vi "AlliGator Calibrate Single Phasor Plot.vi"(0 "Raw Phasor Plot":T6={"Phasor Plot Name"="", "Raw Phasor Plot"=[], "Phasor Frequency"=160000000.0, "[Decay Metadata]"=[], "Raw Phasor Plot SDV"=[], "Phasor SDV Options"={"Compute Estimated SDV"=FALSE, "# Replicas"=100, "Use Estimated Average Phasor"=FALSE}, "[Calibration Phasor]"=[]} {"[Decay Metadata]"."# Folds" min=1; "[Decay Metadata]"."ROI Descriptor"."Contours"."Type" items=["No Selection", "Point", "Line", "Rectangle", "Oval", "Polygon", "Freehand Region", "Annulus", "Unused2", "Unused3", "Broken Line", "Freehand Line", "Rotated Rectangle"]}, 5 "Calibration Phasor":T1, 7 "Calibration Phasor Series":T5, 9 "Phasor Calibration Map":T2={"Phasor Frequency"=80000000.0, "Calibration Lifetime"=1e-09, "ROI Centers"=[], "ROI Descriptors"=[], "Map Resolution X"=0, "Map Resolution Y"=0, "z Array"=[]} {"ROI Descriptors"."Contours"."Type" items=["No Selection", "Point", "Line", "Rectangle", "Oval", "Polygon", "Freehand Region", "Annulus", "Unused2", "Unused3", "Broken Line", "Freehand Line", "Rotated Rectangle"]}, 11 "Error In":errorcluster, 12 "Calibration Map MD5 Digest":string, 13 "Phasor Frequency":dbl[unit]) -> (4 "[Calibrated Phasor]":T4[](array[typedef]), 6 "# Recalibrated Phasors":i32, 8 "[Calibration Phasor]":T1[](array[typedef]), 15 "Error Out":errorcluster)   [LabVIEW 2021, in "AlliGator Phasor Calibration.lvlib"]
doc: "Applies phasor calibration to a single phasor plot.\n\nTakes into account whether a single phasor calibration, a phasor map or a phasor calibration series is used.\n\nFor a calibration map, takes into account the location of each individual phasor in the phasor plot."
uses:
  AlliGator Phasor Calibration.lvlib
  AlliGator Raw Phasor Plot Data v4.ctl
  Phasor/Phasor (g, s).ctl
  AlliGator Decay Metadata v3.ctl
  AlliGator Decay Background Subtraction Info.ctl
  AlliGator Baseline Subtraction Method.ctl
  Graphs/XY Graph/XY Graph Plot Shift Parameters.ctl
  Graphs/XY Graph/XY Graph Plot Shift Method.ctl
  AlliGator Decay Extrapolation Parameters.ctl
  Phasor/Phasor Standard Deviation Options.ctl
  Phasor/Calibration Phasor (m, phi).ctl
  Phasor/Phasor Reference Series.ctl
  Phasor/Phasor Calibration Map v2.ctl
  AlliGator Settings List.ctl
  Phasor/Phasor Calibration Type.ctl
  Utilities/Utilities.lvlib
  Phasor/Phasor.lvlib
  AlliGator Settings.lvlib
  AlliGator Phasor Graph.lvlib
  AlliGator Decay Preprocessing.lvlib
  Graphs/XY Graph/XY Graph Add-Ons.lvlib
panel:
  # "see the AlliGator License on the block diagram (Ctrl+E or Window:Show Block Diagram)"
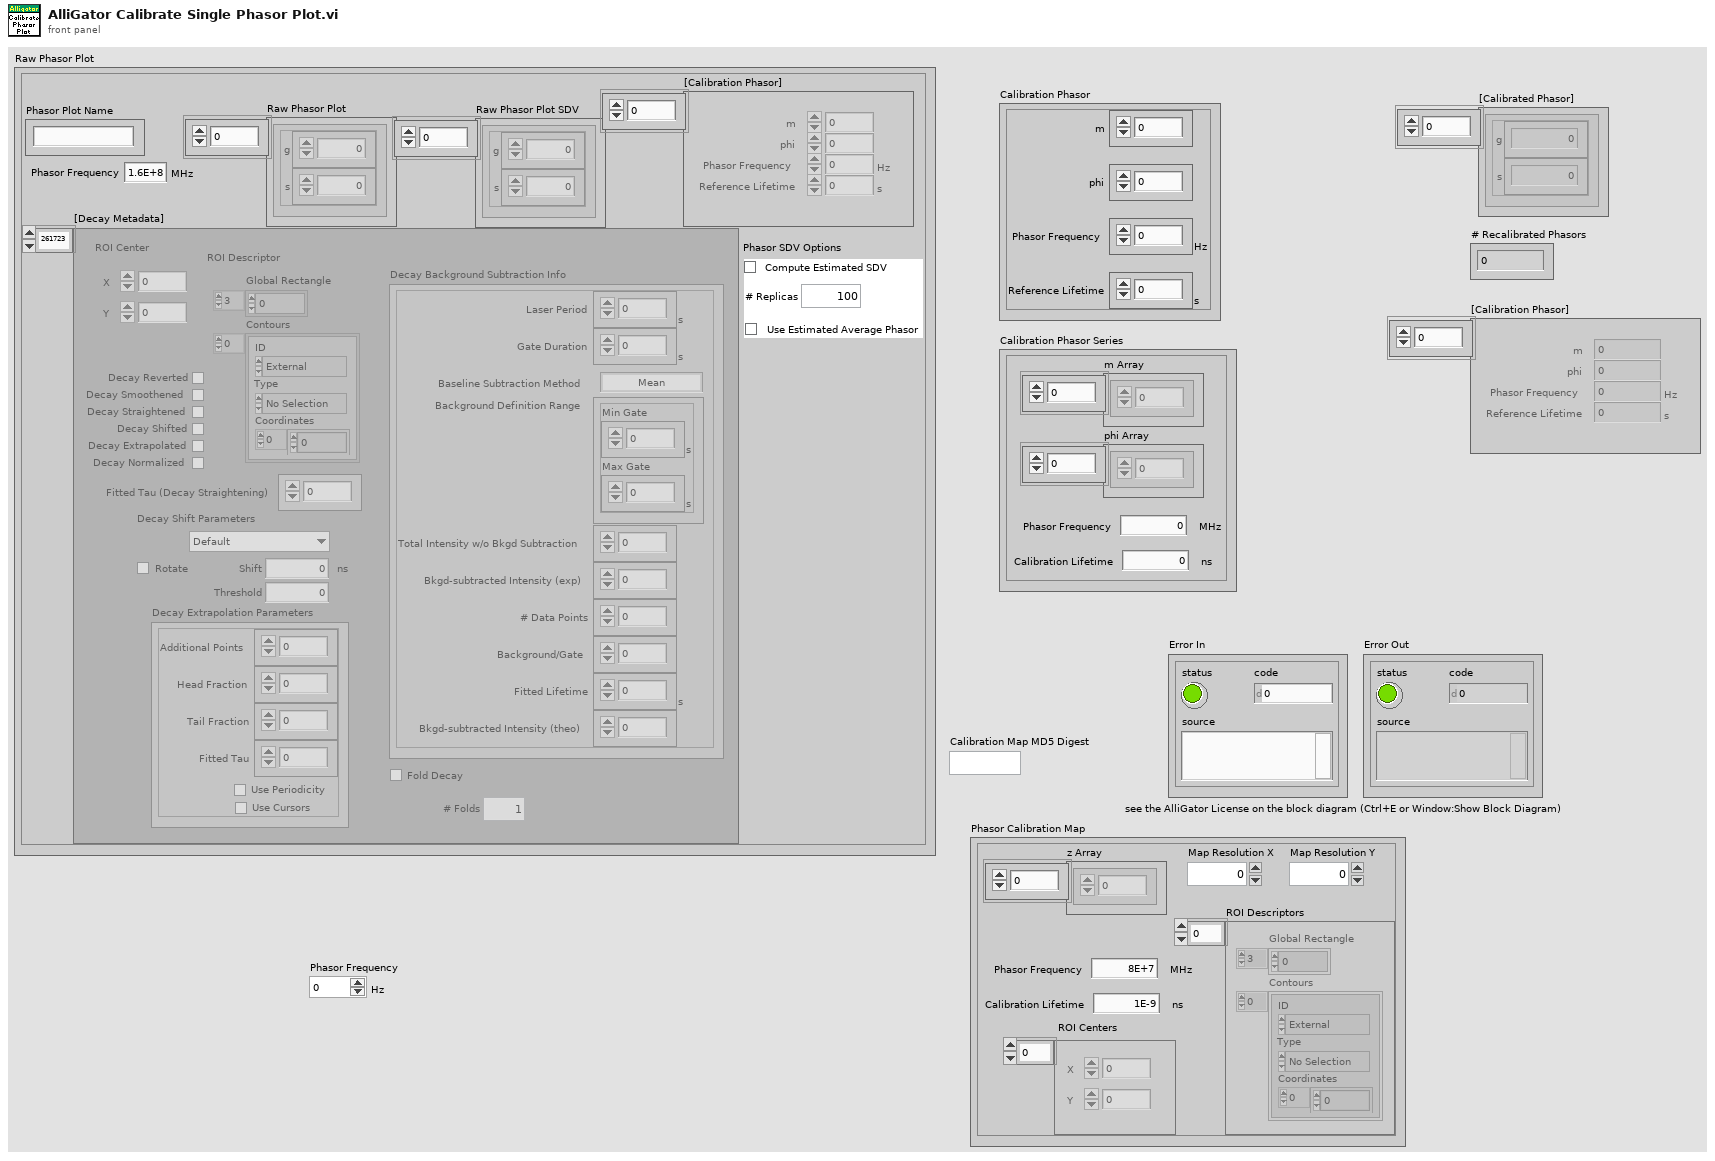
[diagram p1: front panel]
types:
  T1 = typedef "Phasor.lvlib/Calibration Phasor (m, phi).ctl" = cluster{"m":dbl, "phi":dbl, "Phasor Frequency":dbl[unit], "Reference Lifetime":dbl[unit]}
  T2 = typedef "Phasor.lvlib/Phasor Calibration Map v2.ctl" = cluster{"Phasor Frequency":dbl[unit], "Calibration Lifetime":dbl[unit], "ROI Centers":cluster{"X":i32, "Y":i32}[], "ROI Descriptors":T3[], "Map Resolution X":i32, "Map Resolution Y":i32, "z Array":cdb[]}
  T3 = typedef "ROI Descriptor" = cluster{"Global Rectangle":i32[], "Contours":cluster{"ID":enum32{"External", "Internal"}, "Type":u32, "Coordinates":i32[]}[]}
  T4 = typedef "Phasor.lvlib/Phasor (g, s).ctl" = cluster{"g":dbl, "s":dbl}
  T5 = typedef "Phasor.lvlib/Phasor Reference Series.ctl" = cluster{"m Array":dbl[], "phi Array":dbl[], "Phasor Frequency":dbl[unit], "Calibration Lifetime":dbl[unit]}
  T6 = typedef "AlliGator Phasor Graph.lvlib/AlliGator Raw Phasor Plot Data v4.ctl" = cluster{"Phasor Plot Name":string, "Raw Phasor Plot":T4[], "Phasor Frequency":dbl[unit], "[Decay Metadata]":T7[], "Raw Phasor Plot SDV":T4[], "Phasor SDV Options":T13, "[Calibration Phasor]":T1[]}
  T7 = typedef "AlliGator Phasor Graph.lvlib/AlliGator Decay Metadata v3.ctl" = cluster{"ROI Descriptor":T3, "ROI Center":cluster{"X":i32, "Y":i32}, "Decay Background Subtraction Info":T8, "Decay Reverted":bool, "Decay Smoothened":bool, "Decay Straightened":bool, "Fitted Tau (Decay Straightening)":dbl, "Decay Shift Parameters":T10, "Decay Shifted":bool, "Decay Extrapolated":bool, "Decay Extrapolation Parameters":T12, "Decay Normalized":bool, "Fold Decay":bool, "# Folds":u32}
  T8 = typedef "AlliGator Decay Analysis.lvlib/AlliGator Decay Preprocessing.lvlib/AlliGator Decay Background Subtraction Info.ctl" = cluster{"Laser Period":dbl[unit], "Gate Duration":dbl[unit], "Baseline Subtraction Method":T9, "Background Definition Range":cluster{"Min Gate":dbl[unit], "Max Gate":dbl[unit]}, "Total Intensity w/o Bkgd Subtraction":dbl, "Bkgd-subtracted Intensity (exp)":dbl, "# Data Points":i32, "Background/Gate":dbl, "Fitted Lifetime":dbl[unit], "Bkgd-subtracted Intensity (theo)":dbl}
  T9 = typedef "AlliGator Decay Analysis.lvlib/AlliGator Decay Preprocessing.lvlib/AlliGator Baseline Subtraction Method.ctl" = enum16{"Mean", "Min", "Square Gated Single-Exponential", "File", "Constant"}
  T10 = typedef "XY Graph Add-Ons.lvlib/XY Graph Plot Shift Parameters.ctl" = cluster{"Type":T11, "Shift":dbl[unit], "Threshold":dbl, "Rotate":bool}
  T11 = typedef "XY Graph Add-Ons.lvlib/XY Graph Plot Shift Method.ctl" = enum16{"Default", "CFD", "Threshold", "Cross-Correlation"}
  T12 = typedef "AlliGator Decay Analysis.lvlib/AlliGator Decay Preprocessing.lvlib/AlliGator Decay Extrapolation Parameters.ctl" = cluster{"Additional Points":u32, "Head Fraction":dbl, "Fitted Tau":dbl, "Use Periodicity":bool, "Use Cursors":bool, "Tail Fraction":dbl}
  T13 = typedef "Phasor.lvlib/Phasor Standard Deviation Options.ctl" = cluster{"Compute Estimated SDV":bool, "# Replicas":u32, "Use Estimated Average Phasor":bool}
  T14 = typedef "Phasor.lvlib/Phasor Calibration Type.ctl" = enum16{"None", "Single Phasor", "Phasor Series", "Phasor Map"}
  T15 = typedef "AlliGator Settings.lvlib/AlliGator Settings List.ctl" = enum16{"GUI:Visible Settings Tab", "GUI:Last Run Version", "Source Image:Use Image Histogram for Contrast", "Source Image:Low Count Pixels Rejection Options", "Source Image:High Count Pixels Rejection Options", "Source Image:Use Image Brightness", "Source Image:Blend Overlay with Image Background", "Source Image:Use Fixed ROI Diameter", "Source Image:ROI Diameter", "Source Image:ROI Center Color", "Source Image:Peak Threshold", "Source Image:Intensity Threshold", "Source Image:Image Binning Options", "Source Image:Image Smoothing Options", "Source Image:Image Histogram Active", "Source Image:Invert Binary Mask", "Source Image:Hot Pixel Removal", "Source Image:Overlay Analyzed ROI Center", "Source Image:Auto-Adjust Contrast", "Source Image:Histogram Lower Percentile", "Source Image:Histogram Upper Percentile", "Source Image:Save Source Image", "Source Image:Scale Bar Options", "Source Image:Image Resolution (Pixel Size)", "Source Image:Flatfield Correction", "Source Image:Show Dead Left Columns Correction", "Source Image:Dead Left Columns Correction", "Source Image:Image Pre-Processing Operations Order", "Data Information:Gate Width", "Data Information:Nanotime Gate Separation", "Data Information:Macrotime Gate Separation", "Data Information:Gate Step", "Data Information:# Gates", "Data Information:Gate Image Exposure", "Data Information:Gate Image Integration", "Data Information:Gates to Skip", "Data Information:Gates to Keep", "Data Information:Define Gates to", "Data Information:Channel Name", "Data Information:Available Channel Names", "Data Information:Channel Arithmetic", "Data Information:Background File Subtraction", "Data Information:Background File", "Data Information:Background Scaling Factor", "Data Information:Background Pile-up Correction", "Data Information:Background Pixel Well Capacity", "Data Information:Laser Period", "Data Information:SYNC Period", "Data Information:Pile-up Correction", "Data Information:Pixel Well Capacity", "Data Information:Dataset Scaling Factor", "Fluorescence Decay_Decay Pre-Processing:Reverse Gates", "Fluorescence Decay_Decay Pre-Processing:Verbose Decay Pre-Processing", "Fluorescence Decay_Decay Pre-Processing:Use Decay Pre-Processing", "Fluorescence Decay_Decay Pre-Processing:Background Subtraction", "Fluorescence Decay_Decay Pre-Processing:Background Definition Range", "Fluorescence Decay_Decay Pre-Processing:Baseline Subtraction Method", "Fluorescence Decay_Decay Pre-Processing:Decay Pre-Processing Operations Order", "Fluorescence Decay_Decay Pre-Processing:Smoothing Parameter", "Fluorescence Decay_Decay Pre-Processing:Shift Decay", "Fluorescence Decay_Decay Pre-Processing:Decay Shift Parameters", "Fluorescence Decay_Decay Pre-Processing:Fold Decay", "Fluorescence Decay_Decay Pre-Processing:# Folds", "Fluorescence Decay_Decay Pre-Processing:1-Normalize Decay", "Fluorescence Decay_Decay Pre-Processing:[0-1]-Normalize Decay", "Fluorescence Decay_Decay Pre-Processing:Smoothen Decay", "Fluorescence Decay_Decay Pre-Processing:Extrapolate Decay", "Fluorescence Decay_Decay Pre-Processing:Use Periodicity", "Fluorescence Decay_Decay Pre-Processing:Use Cursors", "Fluorescence Decay_Decay Pre-Processing:Tail Fraction", "Fluorescence Decay_Decay Pre-Processing:Head Fraction", "Fluorescence Decay_Decay Pre-Processing:Additional Points", "Fluorescence Decay_Decay Pre-Processing:Straighten Decay", "Fluorescence Decay_Decay Pre-Processing:Constant Background", "Fluorescence Decay_Decay Pre-Processing:Pixel-Normalize Decay", "Fluorescence Decay_Advanced Analysis:Extract IRF instead of Decay", "Fluorescence Decay_Advanced Analysis:IRF Extraction Options", "Fluorescence Decay_Advanced Analysis:IRF Optimization Options", "Fluorescence Decay_Advanced Analysis:Square Pulse Options", "Fluorescence Decay_Advanced Analysis:IRF Order", "Fluorescence Decay_Advanced Analysis:IRF Time Constants", "Fluorescence Decay_Advanced Analysis:Wavelet Analysis Options", "Fluorescence Decay_Advanced Analysis:Average Lifetime Options", "Fluorescence Decay_Fit Options:Fit Options", "Fluorescence Decay_Fit Options:Use Legacy Fitting Approach", "Fluorescence Decay_Fit Options:Use Data Information Laser Period", "Fluorescence Decay_Fit Parameters:Displayed Fit Parameters", "Fluorescence Decay_Fit Parameters:Fit Parameter Constraints", "Fluorescence Decay_Fit Parameters:Export Tabulated Results", "Fluorescence Decay_Fit Parameters:MLE Baseline Offset Type", "Fluorescence Decay_Fit Parameters:MLE Baseline Offset", "Fluorescence Decay_Fit Parameters:Guess Parameter Names", "Fluorescence Decay_Fit Parameters:Guess Parameter Values", "Fluorescence Decay_Fit Parameters:Guess Parameters Options", "Fluorescence Decay_Styles:Show Last Decay Only", "Fluorescence Decay_Styles:Decay Graph Color Array", "Fluorescence Decay:Decay Graph Active", "Fluorescence Decay Statistics:Min Peak Value", "Fluorescence Decay Statistics:Reject Low Decay Peak Pixels", "Fluorescence Decay Statistics:Reject High Decay Peak Pixels", "Fluorescence Decay Statistics:Max Peak Value", "Time Traces:Use File Timestamp", "Time Traces:Time Step", "Time Traces:Use Intensity Correction File", "Time Traces:Intensity Correction File", "Phasor Plot:Phasor Plot Smoothing Options", "Phasor Plot:Phasor Plot Size", "Phasor Plot:Phasor Plot Graphics Options", "Phasor Plot:Cumulative Phasor Plot", "Phasor Plot:Use Phasor Brightness", "Phasor Plot:Blend Overlay with Phasor Background", "Phasor Plot:Save Phasor Plot", "Phasor Plot:Show References", "Phasor Plot:Phasor Ratio Decay Range", "Phasor Plot:Exponential Fading", "Phasor Plot:Phasor Ratio Reference Colors", "Phasor Plot:Reference Radius", "Phasor Plot:Show Color Map Vertices", "Phasor Plot:Phasor Plot Active", "Phasor Plot:Phasor Ratio Color Map Type", "Phasor Plot:Phasor Ratio Color Map", "Phasor Plot:Phasor Ratio Display Range", "Phasor Plot:Selected Image ROI(s)", "Phasor Plot:All Image ROIs", "Phasor Plot:Selected Phasor Plot ROI(s)", "Phasor Plot:All Phasor Plot ROIs", "Phasor Plot:Phasor Ratio Color-Coded Quantity", "Phasor Plot:Store Phasor Harmonics", "Phasor Plot:Draw Reference Segment", "Phasor Plot:User-Defined Quantity", "Phasor Graph:Phasor Frequency", "Phasor Graph:Phasor Ratio Type", "Phasor Graph:Pixel-level Phasor Computation", "Phasor Graph:Save Phasor Graph", "Phasor Graph:Phasor Graph Active", "Phasor Graph:Phasor SDV Options", "Phasor Calibration:Use Backup Calibration if needed", "Phasor Graph:Define Shortest Lifetime as", "Phasor Calibration:Backup Calibration Type", "Phasor Calibration:Calibration Type", "Phasor Calibration:Calibration Lifetime", "Phasor Calibration:Calibration Map Algorithm", "Single-Exponential Phasor Locus (SEPL):Gate Parameters", "Single-Exponential Phasor Locus (SEPL):User-defined Gate", "Single-Exponential Phasor Locus (SEPL):User-defined IRF", "Single-Exponential Phasor Locus (SEPL):Phasor Parameters", "Single-Exponential Phasor Locus (SEPL):Decay & IRF Parameters", "Single-Exponential Phasor Locus (SEPL):Display Parameters", "Lifetime Analysis:Decay Analysis Parameters", "Lifetime Analysis:Lifetime Map Active", "Plugins:Python Settings", "Miscellaneous:Verbose Mode", "Miscellaneous:Beep after Script", "Miscellaneous:Saved Image File Format", "Miscellaneous:Exported Gate Image Settings", "Miscellaneous:Include Loading in Timing", "Miscellaneous:Verbose Settings Mode", "Miscellaneous:Histogram Options", "Miscellaneous:Beep on Error", "Miscellaneous:# Logical Processors Used", "Miscellaneous:ROI Description Max Characters", "Miscellaneous:Verbose Error Mode", "Miscellaneous:Transparent Mask Color"}
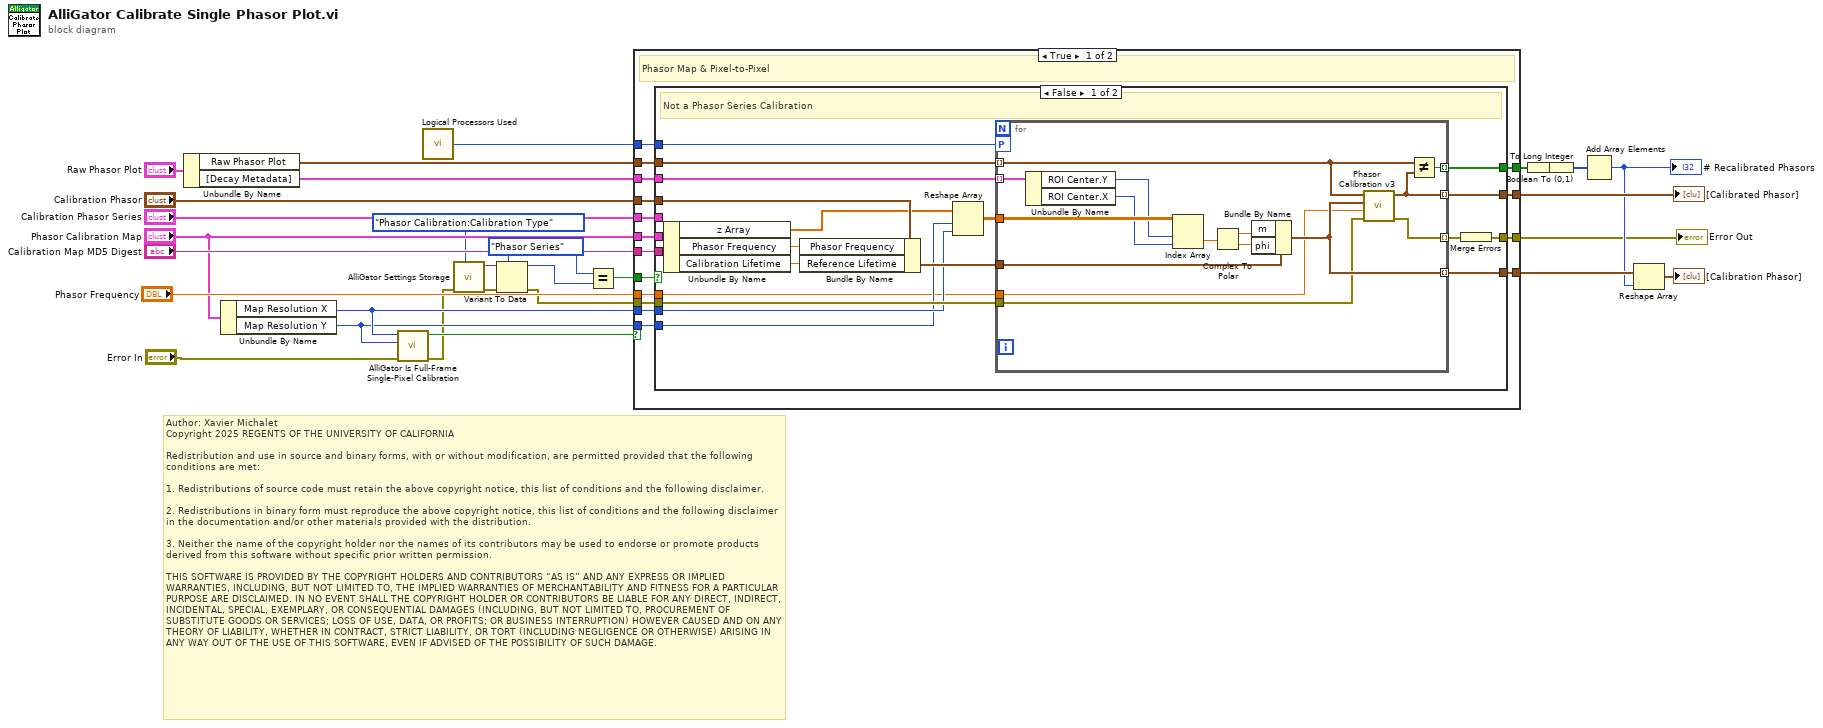
[diagram p0: block diagram]
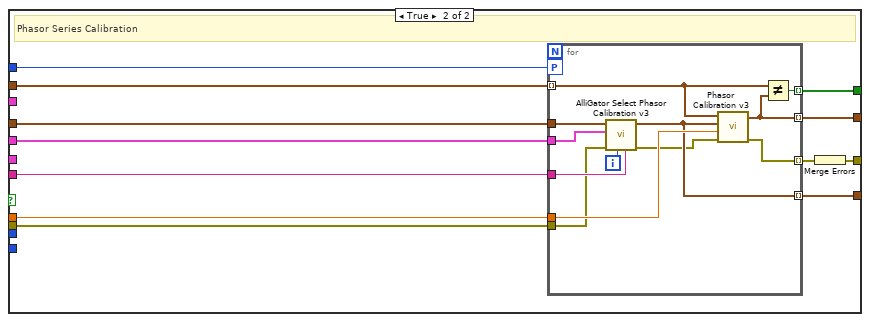
[diagram p2: hidden frame]
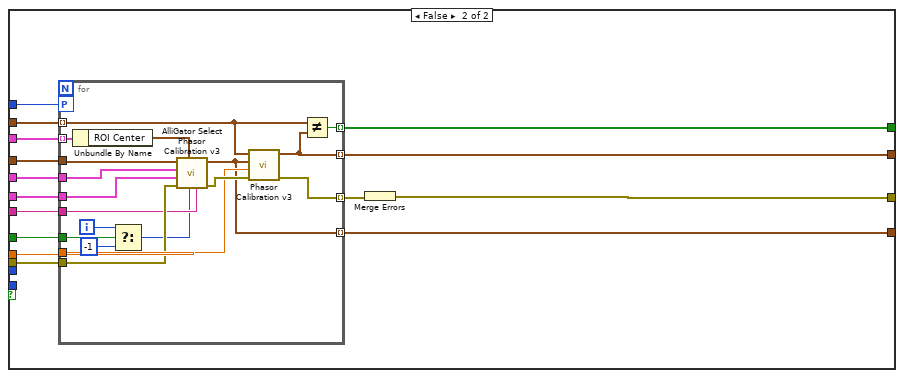
[diagram p3: hidden frame]
diagram:
  w2 = Phasor_Calibration_Type."Phasor Series" ("Calibration Type")
  # "Author: Xavier Michalet\nCopyright 2025 REGENTS OF THE UNIVERSITY OF CALIFORNIA\n\nRedistribution and use in source and binary forms, with or without modification, are permitted provided that the following conditions are met:\n\n1. Redistributions of source code must retain the above copyright notice, this list of conditions and the following disclaimer.\n\n2. Redistributions in binary form must reproduce the above copyright notice, this list of conditions and the following disclaimer in the documentation and/or other materials provided with the distribution.\n\n3. Neither the name of the copyright holder nor the names of its contributors may be used to endorse or promote products derived from this software without specific prior written permission.\n\nTHIS SOFTWARE IS PROVIDED BY THE COPYRIGHT HOLDERS AND CONTRIBUTORS “AS IS” AND ANY EXPRESS OR IMPLIED WARRANTIES, INCLUDING, BUT NOT LIMITED TO, THE IMPLIED WARRANTIES OF MERCHANTABILITY AND FITNESS FOR A PARTICULAR PURPOSE ARE DISCLAIMED. IN NO EVENT SHALL THE COPYRIGHT HOLDER OR CONTRIBUTORS BE LIABLE FOR ANY DIRECT, INDIRECT, INCIDENTAL, SPECIAL, EXEMPLARY, OR CONSEQUENTIAL DAMAGES (INCLUDING, BUT NOT LIMITED TO, PROCUREMENT OF SUBSTITUTE GOODS OR SERVICES; LOSS OF USE, DATA, OR PROFITS; OR BUSINESS INTERRUPTION) HOWEVER CAUSED AND ON ANY THEORY OF LIABILITY, WHETHER IN CONTRACT, STRICT LIABILITY, OR TORT (INCLUDING NEGLIGENCE OR OTHERWISE) ARISING IN ANY WAY OUT OF THE USE OF THIS SOFTWARE, EVEN IF ADVISED OF THE POSSIBILITY OF SUCH DAMAGE."
  n1 = Unbundle By Name("Raw Phasor Plot") -> ("Raw Phasor Plot"=w25:T4[], "[Decay Metadata]"=w24:T7[])
  n2 = Unbundle By Name("Phasor Calibration Map") -> ("Map Resolution X"=w14:i32, "Map Resolution Y"=w11:i32)
  n3 = call "AlliGator Is Full-Frame Single-Pixel Calibration.vi"("error in (no error)"="Error In", "Map Resolution Y"=w11, "Map Resolution X"=w14) -> ("error out"=w5:errorcluster, "Full-Frame Single-Pixel Calibration?"=w12:bool)  [unwired: 7 in]
  n4 = call "Logical Processors Used.vi"() -> ("# Logical Processor Used"=w10:i32)  [unwired: 6 in]
  n5 = call "AlliGator Settings Storage.vi"("AlliGator Settings List"=AlliGator_Settings_List."Phasor Calibration:Calibration Type", "Error In"=w5) -> ("Error Out"=w6:errorcluster, "Variant Data out"=w7:variant)  [unwired: 8 in]
  n6 = Variant To Data(error in=w6, type=w2, Variant=w7) -> (data=w3:T14, error out=w4:errorcluster)
  n7 = Equal?(x=w2, y=w3) -> (x = y?=w1:bool)
  n8 = case shown="True" w12 {
    tunnel: "Calibration Phasor" -> [w39 w118]
    tunnel: "Calibration Phasor Series" -> [w31 w117]
    tunnel: [w45 w116] -> w26
    tunnel: w25 -> [w44 w115]
    tunnel: "Phasor Calibration Map" -> [w43 w114]
    tunnel: w24 -> [w42 w113]
    tunnel: "Calibration Map MD5 Digest" -> [w30 w112]
    tunnel: [w41 w111] -> w22
    tunnel: "Phasor Frequency" -> [w33 w110]
    tunnel: [w40 w109] -> w18
    tunnel: w4 -> [w38 w108]
    tunnel: w14 -> [w37 _]
    tunnel: w11 -> [w36 _]
    tunnel: w10 -> [w35 w107]
    tunnel: [w34 w105] -> w9
    tunnel: w1 -> [w32 w104]
    frame True {
      # "Phasor Map & Pixel-to-Pixel"
      n9 = case shown="False" w32 {
        tunnel: [w64 w91] -> w45
        tunnel: w44 -> [w63 w90]
        tunnel: w43 -> [w62 _]
        tunnel: w42 -> [w61 _]
        tunnel: [w60 w89] -> w41
        tunnel: [w59 w88] -> w40
        tunnel: w39 -> [w58 w81]
        tunnel: w38 -> [w55 w87]
        tunnel: w37 -> [w53 _]
        tunnel: w36 -> [w52 _]
        tunnel: w35 -> [w49 w86]
        tunnel: [w47 w84] -> w34
        tunnel: w33 -> [w46 w83]
        tunnel: w31 -> [_ w82]
        tunnel: w30 -> [_ w80]
        frame False {
          # "Not a Phasor Series Calibration"
          n10 = Unbundle By Name(w62) -> ("z Array"=w54:cdb[], "Phasor Frequency"=w50:dbl[unit], "Calibration Lifetime"=w56:dbl[unit])
          n11 = Bundle By Name(cluster=w58, "Phasor Frequency"=w50, "Reference Lifetime"=w56) -> (w57:T1)
          n12 = Reshape Array(w54, w52, w53) -> (w51:cdb[][])
          n13 = for {
            tunnel: w63 -> [w78] mode=indexing
            tunnel: [w77] -> w64 mode=indexing
            tunnel: w61 -> [w79] mode=indexing
            tunnel: [w75] -> w48 mode=indexing
            workers-P: w49 -> [_]
            tunnel: [w76] -> w60 mode=indexing
            tunnel: [w73] -> w59 mode=indexing
            tunnel: w57 -> [w74]
            tunnel: w46 -> [w72]
            tunnel: w51 -> [w71]
            tunnel: w55 -> [w69]
            n14 = Unbundle By Name(w79) -> ("ROI Center.Y"=w68:i32, "ROI Center.X"=w67:i32)
            n15 = Index Array(array=w71, index (row)=w68, index (col)=w67) -> (element=w70:cdb)
            n16 = Complex To Polar(r * e^(i*theta)=w70) -> (r=w66:dbl, theta=w65:dbl)
            n17 = Bundle By Name(cluster=w74, "m"=w66, "phi"=w65) -> (w73:T1)
            n18 = call "Phasor Calibration v3.vi"("Error In"=w69, "Phasor Frequency"=w72, "Calibration Phasor"=w73, "Measured Phasor"=w78) -> ("Error Out"=w75:errorcluster, "Calibrated Phasor"=w77:T4)  [unwired: 2 in, 4 out]
            n19 = Not Equal?(x=w78, y=w77) -> (x != y?=w76:bool)
          }
          n20 = Merge Errors(w48) -> (w47:errorcluster)
        }
        frame True {
          # "Phasor Series Calibration"
          n21 = for {
            tunnel: w90 -> [w103] mode=indexing
            tunnel: [w102] -> w91 mode=indexing
            tunnel: [w100] -> w85 mode=indexing
            workers-P: w86 -> [_]
            tunnel: [w101] -> w89 mode=indexing
            tunnel: [w94] -> w88 mode=indexing
            tunnel: w83 -> [w99]
            tunnel: w87 -> [w93]
            tunnel: w82 -> [w98]
            tunnel: w81 -> [w97]
            tunnel: w80 -> [w95]
            i -> [w96]
            n22 = call "AlliGator Select Phasor Calibration v3.vi"("Calibration Map MD5 Digest"=w95, "Current Data Set (-1: single)"=w96, "Error In"=w93, "Calibration Phasor Series"=w98, "Calibration Phasor"=w97) -> ("Error Out"=w92:errorcluster, "Calibration Phasor"=w94:T1)  [unwired: 3 in, 2 out]
            n23 = call "Phasor Calibration v3.vi"("Error In"=w92, "Phasor Frequency"=w99, "Calibration Phasor"=w94, "Measured Phasor"=w103) -> ("Error Out"=w100:errorcluster, "Calibrated Phasor"=w102:T4)  [unwired: 2 in, 4 out]
            n24 = Not Equal?(x=w103, y=w102) -> (x != y?=w101:bool)
          }
          n25 = Merge Errors(w85) -> (w84:errorcluster)
        }
      }
    }
    frame False {
      n26 = for {
        tunnel: w115 -> [w129] mode=indexing
        tunnel: w117 -> [w134]
        tunnel: w118 -> [w135]
        tunnel: [w128] -> w116 mode=indexing
        tunnel: w114 -> [w133]
        tunnel: w113 -> [w132] mode=indexing
        tunnel: w108 -> [w136]
        tunnel: [w125] -> w106 mode=indexing
        workers-P: w107 -> [_]
        tunnel: w112 -> [w130]
        tunnel: [w127] -> w111 mode=indexing
        tunnel: w110 -> [w124]
        tunnel: [w123] -> w109 mode=indexing
        tunnel: w104 -> [w119]
        i -> [w122]
        n27 = Unbundle By Name(w132) -> ("ROI Center"=w131:cluster{"X":i32, "Y":i32})
        n28 = Select(t=w122, s=w119, f=-1) -> (s? t:f=w121:i32)
        n29 = call "AlliGator Select Phasor Calibration v3.vi"("Calibration Map MD5 Digest"=w130, "Current Data Set (-1: single)"=w121, "ROI Center (Default: undefined)"=w131, "Error In"=w136, "Phasor Calibration Map"=w133, "Calibration Phasor Series"=w134, "Calibration Phasor"=w135) -> ("Error Out"=w126:errorcluster, "Calibration Phasor"=w123:T1)  [unwired: 1 in, 2 out]
        n30 = call "Phasor Calibration v3.vi"("Error In"=w126, "Phasor Frequency"=w124, "Calibration Phasor"=w123, "Measured Phasor"=w129) -> ("Error Out"=w125:errorcluster, "Calibrated Phasor"=w128:T4)  [unwired: 2 in, 4 out]
        n31 = Not Equal?(x=w129, y=w128) -> (x != y?=w127:bool)
      }
      n32 = Merge Errors(w106) -> (w105:errorcluster)
    }
  }
  "Error Out" <- w9
  "[Calibrated Phasor]" <- w26
  n33 = Boolean To (0,1)(Boolean=w22) -> (0, 1=w21:i16[])
  n34 = To Long Integer(number=w21) -> (32bit integer=w20:i32[])
  n35 = Add Array Elements(numeric array=w20) -> (sum=w17:i32)
  "# Recalibrated Phasors" <- w17
  n36 = Reshape Array(w18, w17) -> (→"[Calibration Phasor]":T1[])
